vi "PIDF Test.vi"() -> ()   [LabVIEW 2016]
panel:
  out "Waveform Chart":T1(graph)={"setpoint"=20.0, "output"=7.6923076923077005, "Plant Output"=19.23076923076923}
  in  "stop":bool
  in  "PIDF gains":cluster{"Kp":dbl, "Ki":dbl, "Kd":dbl, "Kf":dbl}={"Kp"=10.0, "Ki"=100.0, "Kd"=0.0, "Kf"=0.0} {"Kf" format="%.3f"; "Kd" format="%.3f"; "Ki" format="%.3f"; "Kp" format="%.3f"}
  in  "setpoint":dbl=20.0 format="%.2f"
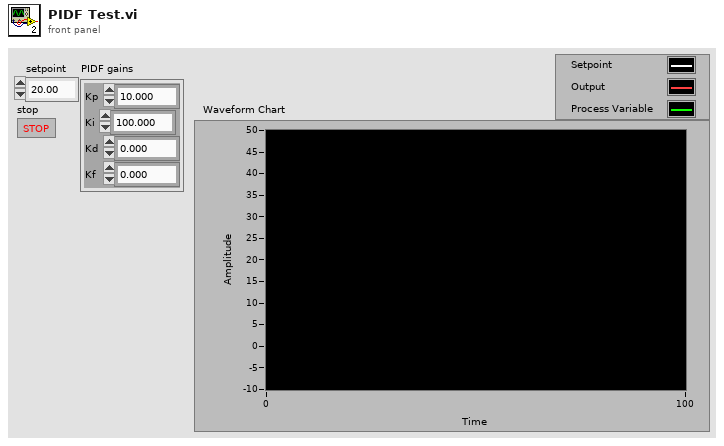
[diagram p1: front panel]
types:
  T1 = cluster{"setpoint":dbl, "output":dbl, "Plant Output":dbl}
  T2 = cluster{"static gain":dbl, "lag (s)":dbl, "deadtime (s)":dbl, "load":dbl, "deadband":dbl, "sensor noise":dbl, "initial PV":dbl, "plant noise":dbl}
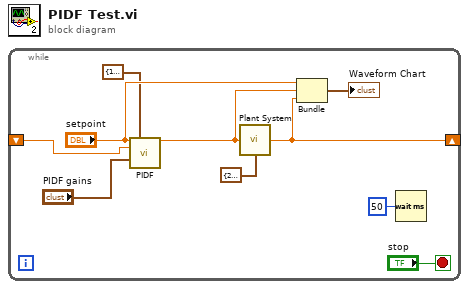
[diagram p0: block diagram]
diagram:
  n1 = while {
    shift-right: [w4] -> _
    shift-left: _ -> [w8]
    stop <- "stop" stop-if-true
    n2 = call "PIDF.vi"("setpoint"="setpoint", "output range"=cluster{"output high":dbl, "output low":dbl} {"output high"=10.0, "output low"=-10.0}, "process variable"=w8, "PIDF gains"="PIDF gains") -> ("output"=w3:dbl)  [unwired: 11 in]
    n3 = call "Plant System.vi"("Plant Input"=w3, "process parameters"=T2 {"static gain"=2.5, "lag (s)"=2.5, "deadtime (s)"=0.001, "load"=0.0, "deadband"=0.0, "sensor noise"=0.0, "initial PV"=30.0, "plant noise"=0.0}) -> ("Plant Output"=w4:dbl)  [unwired: 13 in]
    n4 = Bundle("setpoint"="setpoint", "output"=w3, "Plant Output"=w4) -> (→"Waveform Chart":T1)  [unwired: 1 in]
    n5 = Wait (ms)(milliseconds to wait=u32 50) -> ()  [unwired: 1 out]
  }
